vi "GLOBAL_Scaler_Rate.vi"(3 "Data in":dbl[](array[numeric]), 5 "State":enum16{"Initialise", "Write", "Read"}(ring)) -> (0 "Valid Read?":bool, 1 "Data out":dbl[](array[numeric]))   [LabVIEW 2014]
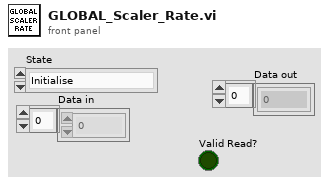
[diagram p1: front panel]
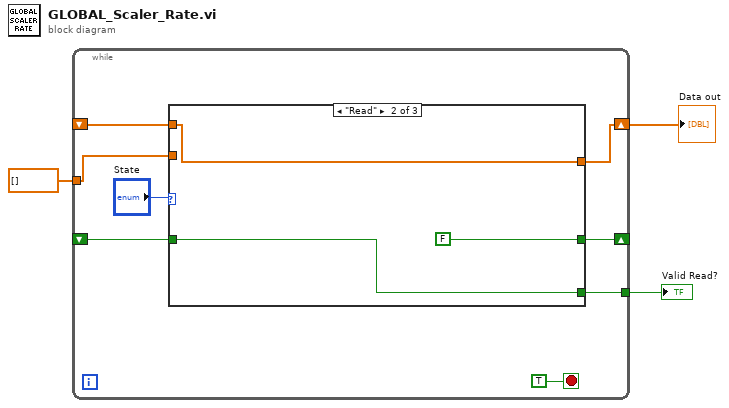
[diagram p0: block diagram]
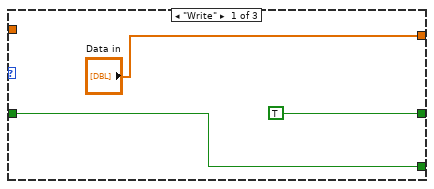
[diagram p2: hidden frame]
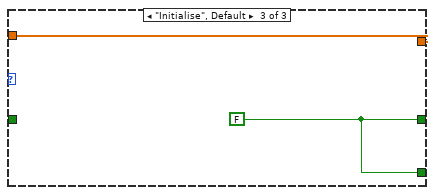
[diagram p3: hidden frame]
diagram:
  n1 = while {
    shift-right: [w7] -> w3
    shift-left: _ -> [w9]
    tunnel: dbl[] [] ("Data in") -> [w8]
    shift-right: [w4] -> _
    shift-left: _ -> [w6]
    tunnel: [w5] -> w1
    stop <- TRUE stop-if-true
    n2 = case shown="\"Read\"" "State" {
      tunnel: ["Data in" w17 w19] -> w7
      tunnel: w9 -> [_ w17 _]
      tunnel: w8 -> [_ _ w19]
      tunnel: [TRUE FALSE w18] -> w4
      tunnel: w6 -> [w12 w16 _]
      tunnel: [w12 w16 w18] -> w5
      frame "Write" {
      }
      frame "Read" {
      }
      frame "Initialise", Default {
        w18 = FALSE
      }
    }
  }
  "Data out" <- w3
  "Valid Read?" <- w1
